vi "removeItem.vi"(8 "error in (no error)":errorcluster, 10 "Key":string, 11 "Bucket in":refnum<class "Bucket.lvclass">) -> (0 "error out":errorcluster, 3 "Bucket out":refnum<class "Bucket.lvclass">)   [LabVIEW 2017, in "Bucket.lvclass"]
uses:
  <userlib>/836-Library/Data_Structures/Bucket/Bucket.lvclass
  <userlib>/836-Library/Data_Structures/Bucket/Bucket.lvclass/Bucket.ctl
  <userlib>/836-Library/Data_Structures/Bucket/Types/KeyValuePair.ctl
  <vilib>/Utility/error.llb/Error Cluster From Error Code.vi
  <vilib>/ErrorRing/Error Ring.xnode
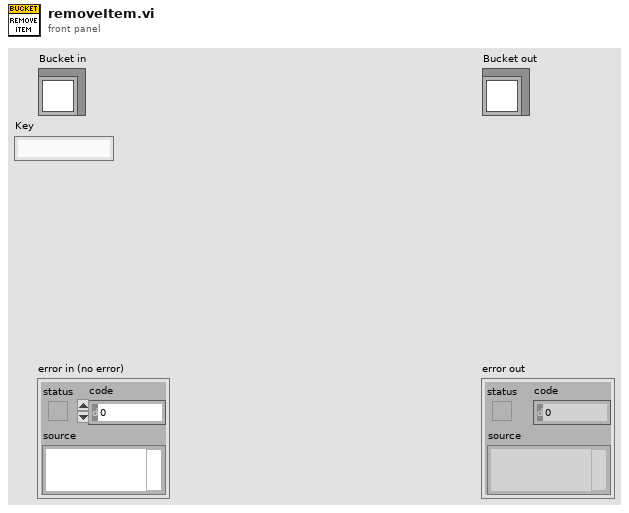
[diagram p1: front panel]
types:
  T1 = typedef "KeyValuePair.ctl" = cluster{"Key":string, "Value":variant}
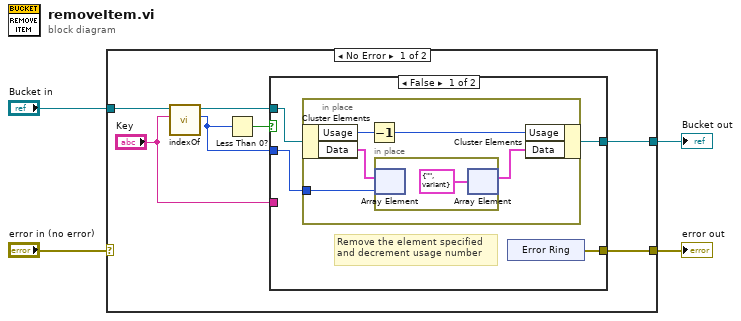
[diagram p0: block diagram]
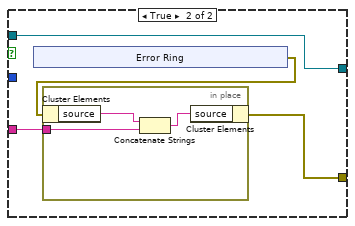
[diagram p2: hidden frame]
diagram:
  n1 = case shown="No Error" "error in (no error)" {
    selector: "error in (no error)" -> [_ w36]
    tunnel: [w5 w36] -> w3
    tunnel: [w7 w35] -> w1
    tunnel: "Bucket in" -> [w11 w35]
    frame No Error {
      n2 = call <userlib>:"indexOf.vi"("Key"="Key", "Bucket in"=w11) -> ("Index"=w8:i32, "Bucket out"=w10:refnum<class "Bucket.lvclass">)  [unwired: 7 in, 1 out]
      n3 = Less Than 0?(x=w8) -> (x < 0?=w9:bool)
      n4 = case shown="False" w9 {
        tunnel: w10 -> [w15 w26]
        tunnel: w8 -> [w14 _]
        tunnel: [w13 w26] -> w7
        tunnel: "Key" -> [_ w24]
        tunnel: [w12 w23] -> w5
        frame False {
          # "Remove the element specified\nand decrement usage number"
          n5 = in-place {
            in-place-border: w14 -> [w18]
            n6 = in-place-cluster #1(w15) -> ("Usage"=w20:u32, "Data"=w19:T1[])
            n7 = Decrement(x=w20) -> (x-1=w21:u32)
            n8 = in-place {
              n9 = in-place-array #2(w19, w18) -> ()  [unwired: 1 out]
              n10 = in-place-array #2(T1 {"Key"="", "Value"=variant} ("element")) -> (w17:T1[])  [unwired: 1 out]
            }
            n11 = in-place-cluster #1("Usage"=w21, "Data"=w17) -> (w13:refnum<class "Bucket.lvclass">)
          }
          n12 = xnode "Error Ring"() -> ("error out"=w12:errorcluster)
        }
        frame True {
          n13 = xnode "Error Ring"() -> ("error out"=w25:errorcluster)
          n14 = in-place {
            in-place-border: w24 -> [w27]
            n15 = in-place-cluster #3(w25) -> ("source"=w28:string)
            n16 = Concatenate Strings(w28, w27) -> (w29:string)
            n17 = in-place-cluster #3("source"=w29) -> (w23:errorcluster)
          }
        }
      }
    }
    frame Error {
    }
  }
  "error out" <- w3
  "Bucket out" <- w1
